vi "LC1-to-newtons.vi"(11 "LC In":dbl) -> (3 "Newtons Out":dbl)   [LabVIEW 2025]
uses:
  <vilib>/express/express arith-compare/Formula/XNode/ExpressFormulaBlockNode.xnode
  <vilib>/ptbypt/NI_PtbyPt.lvlib
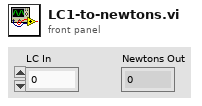
[diagram p1: front panel]
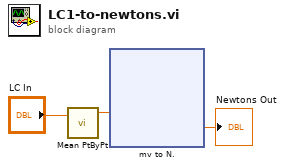
[diagram p0: block diagram]
diagram:
  n1 = call <vilib>:"Mean PtByPt.vi"("x"="LC In") -> ("mean"=w1:dbl)  [unwired: 3 in, 1 out]
  n2 = xnode ("mv to N.")("mv"=w1) -> ("Result"=→"Newtons Out":dbl)  [unwired: 1 in, 1 out]
